vi "AB_860_900_Project_Destinations.vi"(6 "ProjectPath":path, 7 "action":T3, 8 "error in (no error)":errorcluster, 9 "index":i32, 10 "data in":T2, 11 "buildObject":T1) -> (0 "error out":errorcluster, 1 "index out":i32, 2 "data out":T2, 3 "buildObject out":T1)   [LabVIEW 2020]
doc: "Reads and writes the data to the object property bag."
uses:
  <resource>/Framework/Providers/API/ItemRef.ctl
  <vilib>/AppBuilder/RW_Project/AB_RW_Project_PropBag_Action.ctl
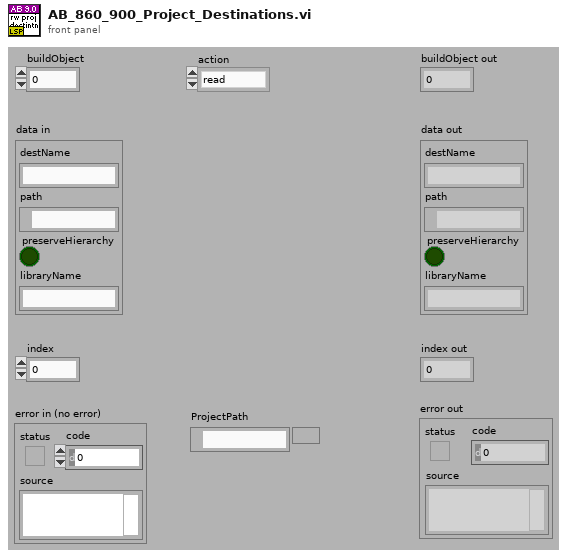
[diagram p1: front panel]
types:
  T1 = typedef "ItemRef.ctl" = u64
  T2 = cluster{"destName":string, "path":path, "preserveHierarchy":bool, "libraryName":string}
  T3 = typedef "AB_RW_Project_PropBag_Action.ctl" = enum16{"read", "write", "clear", "readPrevious", "writePrevious", "clearPrevious"}
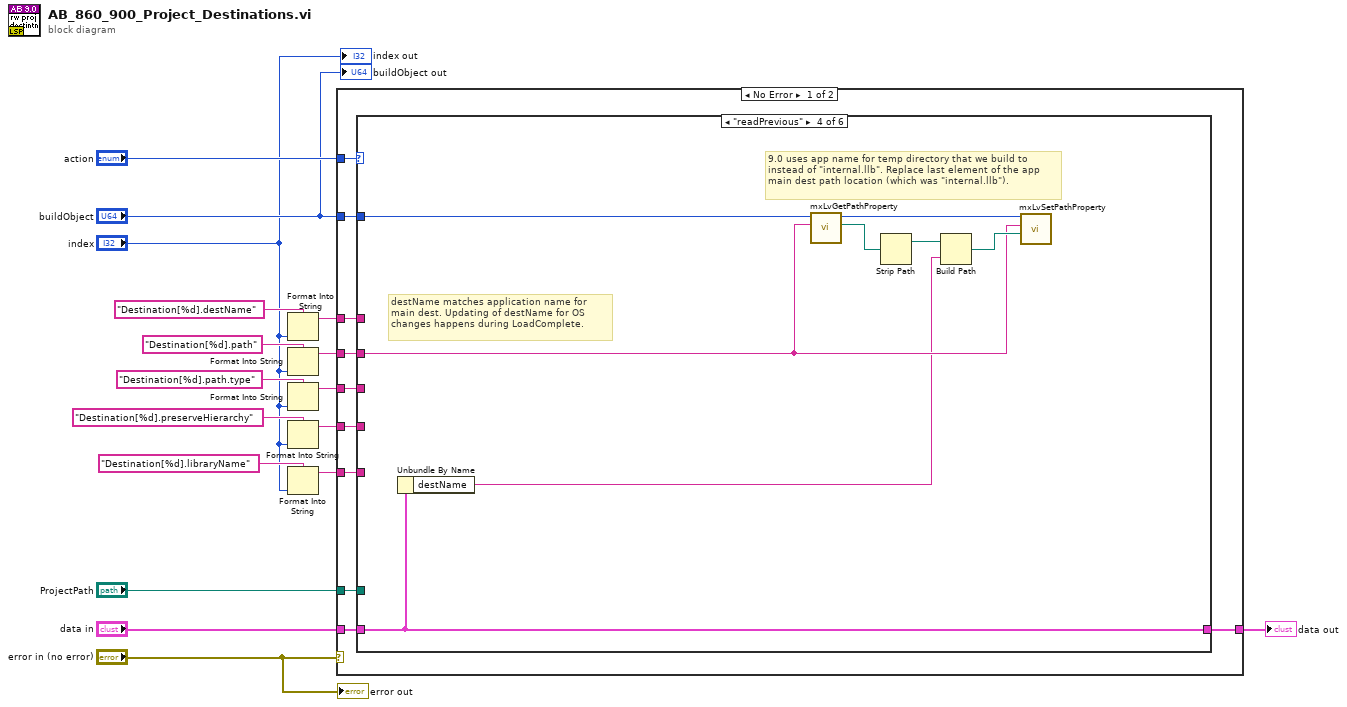
[diagram p0: block diagram]
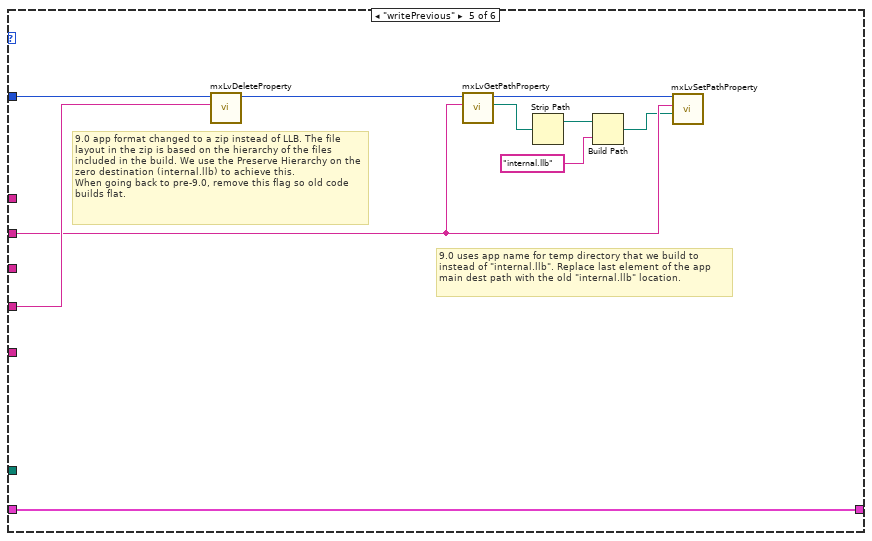
[diagram p5: hidden frame]
diagram:
  n1 = Format Into String(format string="Destination[%d].destName", "index") -> (resulting string=w14:string)  [unwired: 2 in, 1 out]
  n2 = Format Into String(format string="Destination[%d].path", "index") -> (resulting string=w11:string)  [unwired: 2 in, 1 out]
  n3 = Format Into String(format string="Destination[%d].path.type", "index") -> (resulting string=w10:string)  [unwired: 2 in, 1 out]
  n4 = Format Into String(format string="Destination[%d].preserveHierarchy", "index") -> (resulting string=w4:string)  [unwired: 2 in, 1 out]
  n5 = Format Into String(format string="Destination[%d].libraryName", "index") -> (resulting string=w3:string)  [unwired: 2 in, 1 out]
  n6 = case shown="No Error" "error in (no error)" {
    tunnel: "action" -> [w27 _]
    tunnel: "data in" -> [w26 w50]
    tunnel: w14 -> [w25 _]
    tunnel: w11 -> [w24 _]
    tunnel: w10 -> [w23 _]
    tunnel: [w22 w50] -> w9
    tunnel: "buildObject" -> [w21 _]
    tunnel: "ProjectPath" -> [w20 _]
    tunnel: w4 -> [w19 _]
    tunnel: w3 -> [w18 _]
    frame No Error {
      n7 = case shown="\"readPrevious\"" w27 {
        tunnel: w21 -> [_ _ _ w31 w47 _]
        tunnel: w26 -> [w28 w29 w30 w33 w48 w49]
        tunnel: w25 -> [_ _ _ _ _ _]
        tunnel: w24 -> [_ _ _ w34 w45 _]
        tunnel: w23 -> [_ _ _ _ _ _]
        tunnel: [w28 w29 w30 w33 w48 w49] -> w22
        tunnel: w20 -> [_ _ _ _ _ _]
        tunnel: w19 -> [_ _ _ _ w46 _]
        tunnel: w18 -> [_ _ _ _ _ _]
        frame "read" {
        }
        frame "write" {
        }
        frame "clear" {
        }
        frame "readPrevious" {
          # "destName matches application name for main dest. Updating of destName for OS changes happens during LoadComplete."
          # "9.0 uses app name for temp directory that we build to  instead of \"internal.llb\". Replace last element of the app main dest path location (which was \"internal.llb\")."
          n8 = Unbundle By Name(w33) -> ("destName"=w32:string)
          n9 = call <resource>:"mxLvGetPathProperty.vi"("Tag"=w34, "Item"=w31) -> ("Path"=w35:path, "Item"=w38:T1)  [unwired: 2 in, 6 out]
          n10 = Strip Path(path=w35) -> (stripped path=w36:path)  [unwired: 1 out]
          n11 = Build Path(base path=w36, name or relative path=w32) -> (appended path=w37:path)
          n12 = call <resource>:"mxLvSetPathProperty.vi"("Path"=w37, "Tag"=w34, "Item"=w38) -> ()  [unwired: 2 in, 7 out]
        }
        frame "writePrevious" {
          # "9.0 uses app name for temp directory that we build to  instead of \"internal.llb\". Replace last element of the app main dest path with the old \"internal.llb\" location."
          # "9.0 app format changed to a zip instead of LLB. The file layout in the zip is based on the hierarchy of the files included in the build. We use the Preserve Hierarchy on the zero destination (internal.llb) to achieve this. \nWhen going back to pre-9.0, remove this flag so old code builds flat."
          n13 = call <resource>:"mxLvDeleteProperty.vi"("Tag"=w46, "Item"=w47) -> ("Item"=w40:T1)  [unwired: 1 in, 8 out]
          n14 = call <resource>:"mxLvGetPathProperty.vi"("Tag"=w45, "Item"=w40) -> ("Path"=w44:path, "Item"=w41:T1)  [unwired: 2 in, 6 out]
          n15 = Strip Path(path=w44) -> (stripped path=w43:path)  [unwired: 1 out]
          n16 = Build Path(base path=w43, name or relative path="internal.llb") -> (appended path=w42:path)
          n17 = call <resource>:"mxLvSetPathProperty.vi"("Path"=w42, "Tag"=w45, "Item"=w41) -> ()  [unwired: 2 in, 7 out]
        }
        frame "clearPrevious" {
        }
      }
    }
    frame Error {
    }
  }
  "data out" <- w9
  "error out" <- "error in (no error)"
  "buildObject out" <- "buildObject"
  "index out" <- "index"
